vi "FTW-ProjectManager-SaveProject.vi"(0 "Project Manager":refnum<class "FTW-ProjectManager.lvclass">, 11 "error in":errorcluster) -> (4 "Project Manager out":refnum<class "FTW-ProjectManager.lvclass">, 15 "error out":errorcluster)   [LabVIEW 2012, in "FTW-ProjectManager.lvclass"]
uses:
  FTW-ProjectManager.lvclass
  FTW-ProjectManager.lvclass/FTW-ProjectManager.ctl
panel:
  # "Inputs"
  # "Outputs"
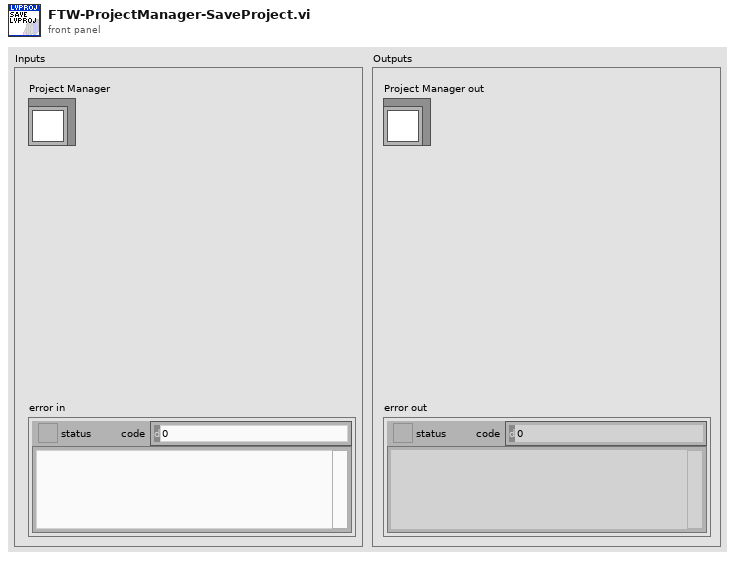
[diagram p1: front panel]
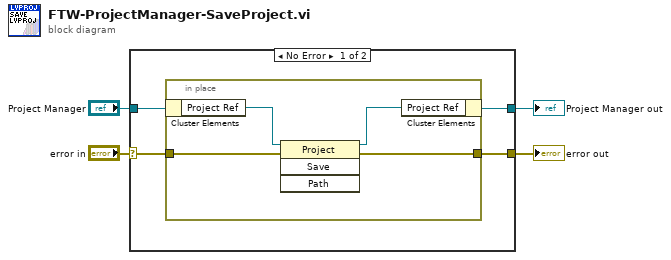
[diagram p0: block diagram]
diagram:
  n1 = case shown="No Error" "error in" {
    selector: "error in" -> [w8 w14]
    tunnel: [w7 w14] -> w4
    tunnel: [w5 w13] -> w2
    tunnel: "Project Manager" -> [w6 w13]
    frame No Error {
      n2 = in-place {
        in-place-border: w8 -> [w12]
        in-place-border: [w11] -> w7
        n3 = in-place-cluster #1(w6) -> ("Project Ref"=w10:refnum<vi>)
        n4 = invoke class="Project" method="Save"(reference=w10, error in=w12) -> (reference out=w9:refnum<vi>, error out=w11:errorcluster)  [unwired: 2 in, 2 out]
        n5 = in-place-cluster #1("Project Ref"=w9) -> (w5:refnum<class "FTW-ProjectManager.lvclass">)
      }
    }
    frame Error {
    }
  }
  "error out" <- w4
  "Project Manager out" <- w2
